vi "Get_Devices.vi"(8 "error in (no error)":errorcluster) -> (0 "error out":errorcluster, 2 "devices":T1(array[cluster]))   [LabVIEW 2019]
uses:
  <vilib>/Utility/error.llb/Error Cluster From Error Code.vi
  <vilib>/ErrorRing/Error Ring.xnode
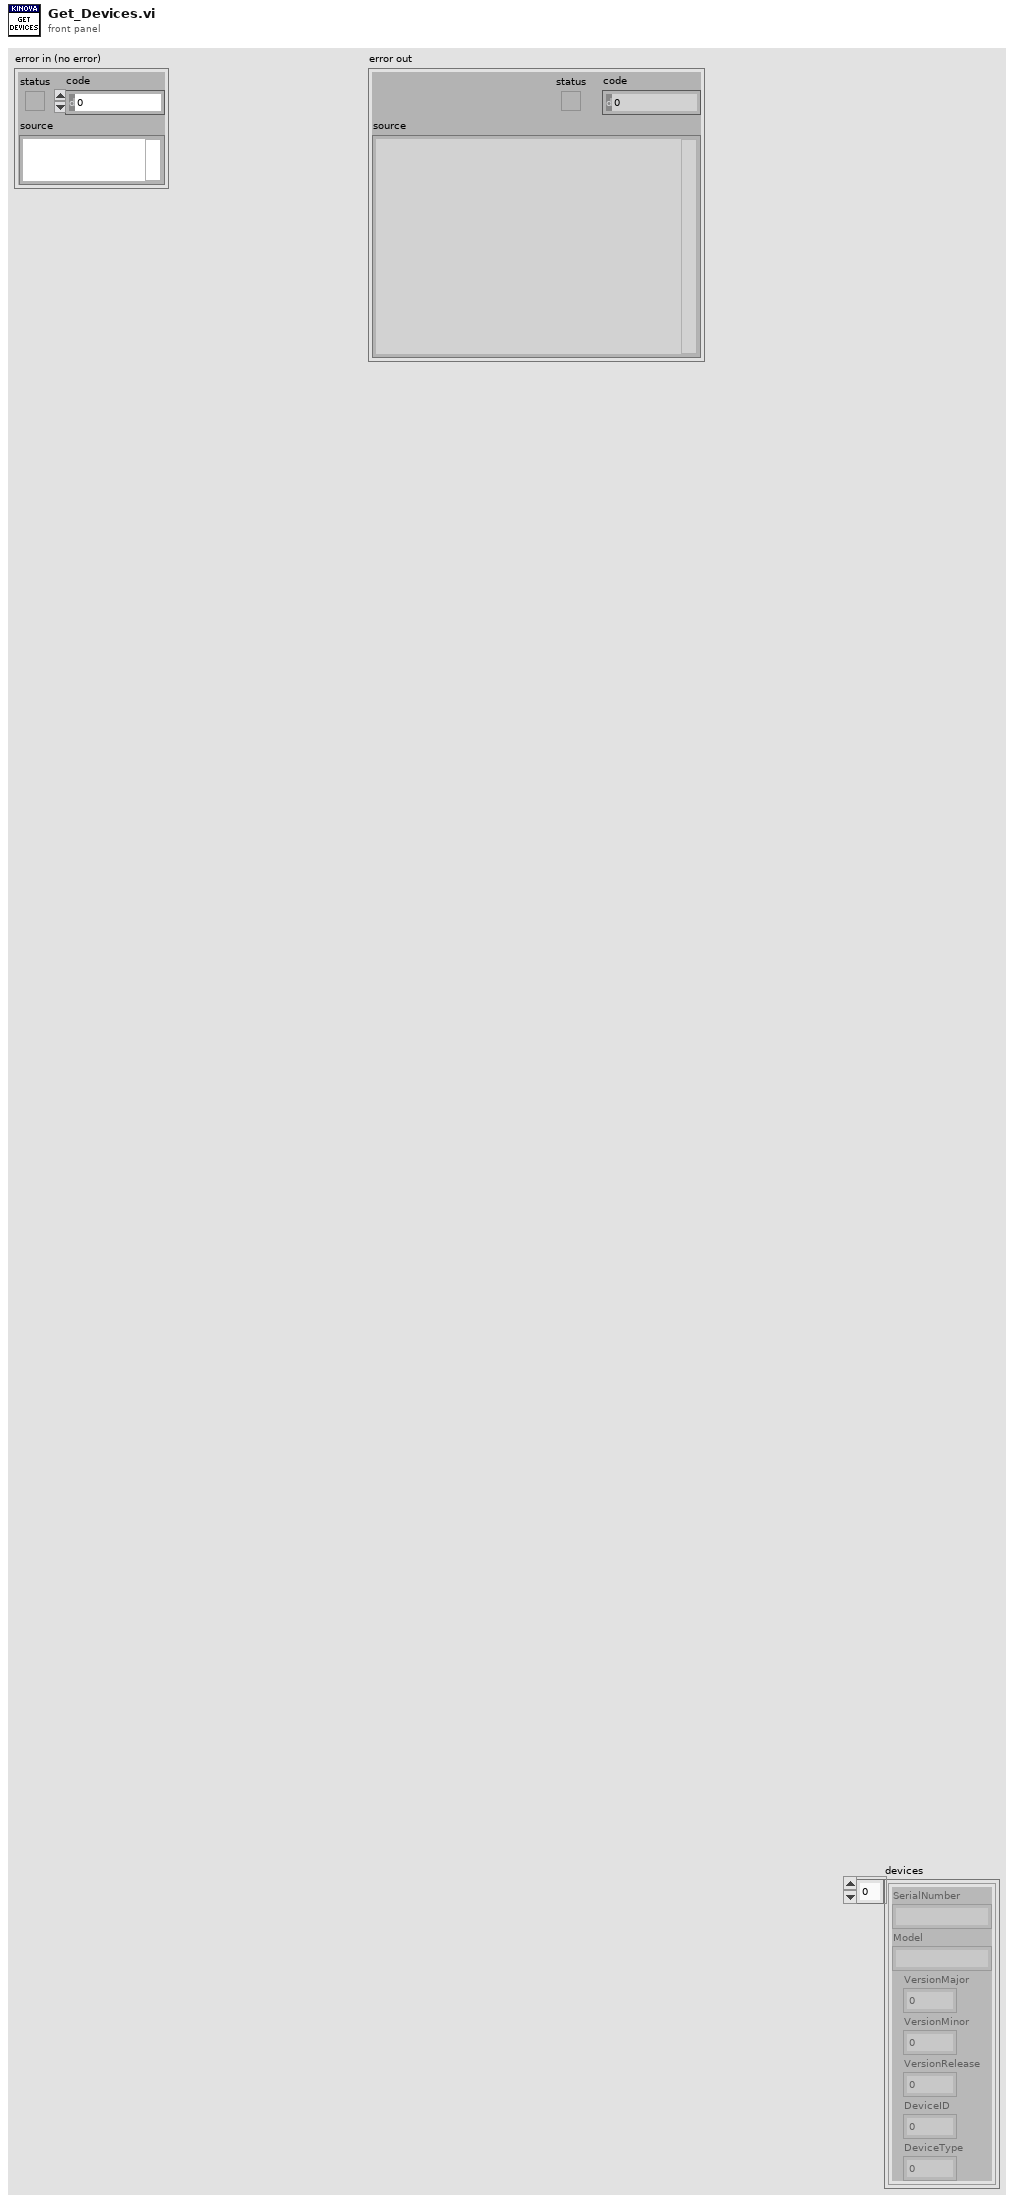
[diagram p1: front panel]
types:
  T1 = cluster{"SerialNumber":string, "Model":string, "VersionMajor":i32, "VersionMinor":i32, "VersionRelease":i32, "DeviceID":i32, "DeviceType":i32}[]
  T2 = cluster{"SerialNumber":string, "Model":string, "VersionMajor":i32, "VersionMinor":i32, "VersionRelease":i32, "DeviceID":i32, "DeviceType":i32}
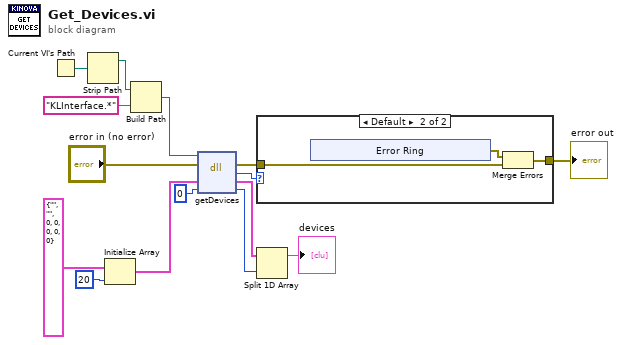
[diagram p0: block diagram]
diagram:
  n1 = Current VI's Path() -> (path=w13:path)
  n2 = Strip Path(path=w13) -> (stripped path=w12:path)  [unwired: 1 out]
  n3 = Initialize Array(T2 {"SerialNumber"="", "Model"="", "VersionMajor"=0, "VersionMinor"=0, "VersionRelease"=0, "DeviceID"=0, "DeviceType"=0} ("Kinova Device"), 20 ("dimension size")) -> (w7:T1)
  n4 = Build Path(base path=w12, name or relative path="KLInterface.*") -> (appended path=w1:path)
  n5 = dll-call lib="C:/Users/mcjssdcc/source/repos/Kinova Labview Interface/Debug/KLInterface.dll" fn="getDevices"(path in=w1, error in="error in (no error)", "devices"=w7, "devicecount"=0) -> (error out=w11:errorcluster, "return type"=w9:i32, "devices"=w4:T1, "devicecount"=w5:i32)  [unwired: 1 in, 1 out]
  n6 = case shown="Default" w9 {
    tunnel: [w16 w18] -> w10
    tunnel: w11 -> [w16 w17]
    frame 1 {
    }
    frame Default {
      n7 = xnode "Error Ring"() -> ("error out"=w19:errorcluster)
      n8 = Merge Errors(w19, w17) -> (w18:errorcluster)
    }
  }
  "error out" <- w10
  n9 = Split 1D Array(array=w4, index=w5) -> (first subarray=→"devices":T1)  [unwired: 1 out]
